vi "knob global.vi"() -> ()   [LabVIEW 2015]
panel:
  in  "Knob type":string="Phidgets 3-axis USB knob box"
  in  "Encoder resolution (1/turn)":dbl=80.0
  in  "Serial numbers":i32[](array[numeric])=[82255, 82264, 82265]
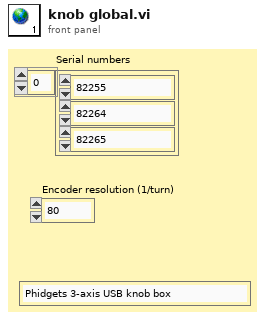
[diagram p1: front panel]
diagram:
